vi "set stage speeds.vi"() -> ()   [LabVIEW 2012]
uses:
  GFG/GFGnumericGet.vi
  GFG/GFG library.lvlib
panel:
  in  "fast":dbl
  in  "slow":dbl
  in  "OK Button":bool
  # "Set stage speed (arbitrary units)"
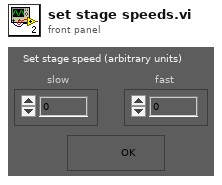
[diagram p1: front panel]
types:
  T1 = enum32{"Invalid", "Standard", "Closed", "Hidden", "Minimized", "Maximized"}
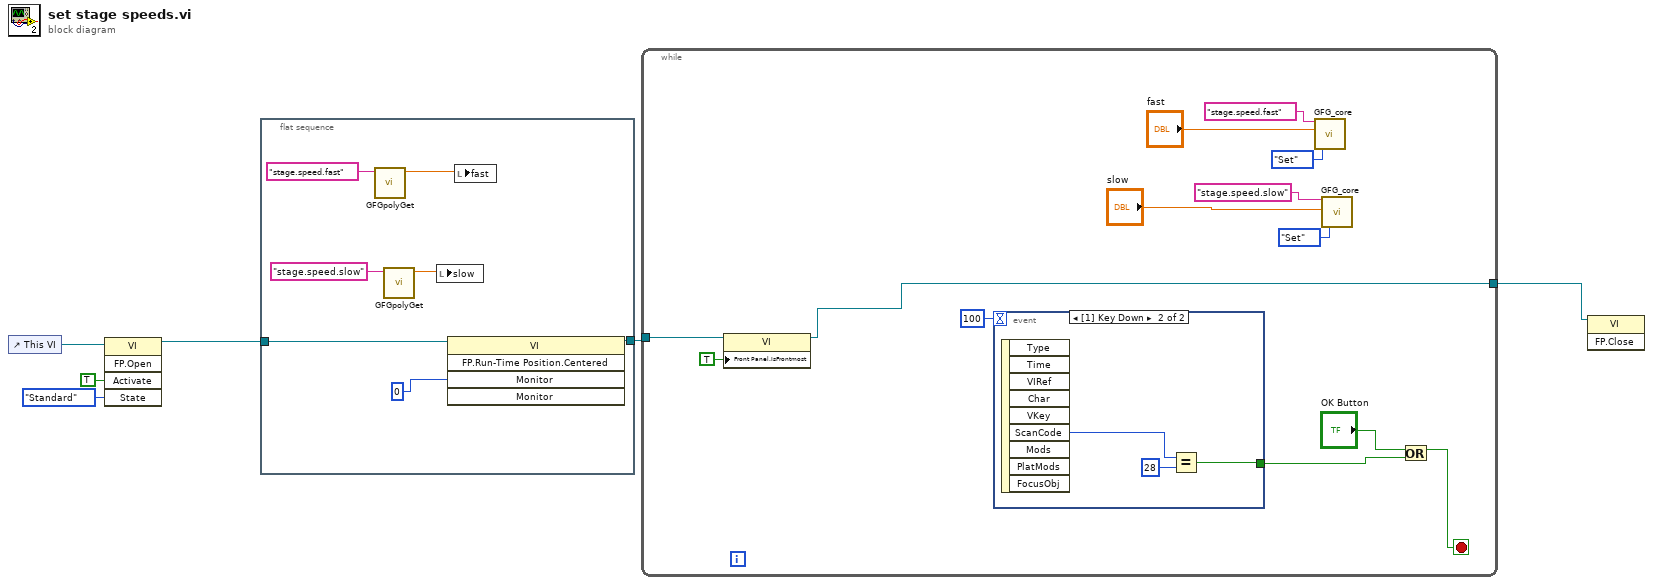
[diagram p0: block diagram]
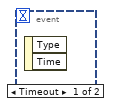
[diagram p2: hidden frame]
diagram:
  n1 = control-ref of="This VI"() -> (w4:refnum<vi>)
  n2 = invoke class="VI" method="FP.Open"(reference=w4, "Activate"=TRUE ("Activate?"), "State"=T1."Standard") -> (reference out=w1:refnum<vi>)  [unwired: 2 in, 4 out]
  n3 = flat-sequence {
    tunnel: [w12] -> w2
    tunnel: w1 -> [w11]
    frame #0 {
      n4 = call-poly "GFGpolyGet.vi"("Variable Name in"="stage.speed.fast") -> ("Numeric"=w8:dbl)  [unwired: 9 in, 1 out]
      n5 = call-poly "GFGpolyGet.vi"("Variable Name in"="stage.speed.slow") -> ("Numeric"=w7:dbl)  [unwired: 9 in, 1 out]
      n6 = local write "slow"(w7) -> ()
      n7 = invoke class="VI" method="FP.Run-Time Position.Centered"(reference=w11, "Monitor"=i16 0) -> (reference out=w12:refnum<vi>)  [unwired: 3 in, 4 out]
      n8 = local write "fast"(w8) -> ()
    }
  }
  n9 = while {
    tunnel: w2 -> [w23]
    tunnel: [w22] -> w3
    stop <- w21 stop-if-true
    n10 = property class="VI"(reference=w23, "Front Panel.IsFrontmost"=TRUE ("Front Panel Window:Is Frontmost")) -> (reference out=w22:refnum<vi>)  [unwired: 1 in, 1 out]
    n11 = event shown="[1] Key Down" {
      selector: _ -> [_ _]
      dyn-events: _ -> [_ _]
      timeout: 100 -> [_ _]
      tunnel: [_ w27] -> w20
      event Timeout {
        n12 = event-data() -> ()  [unwired: 1 in, 2 out]
      }
      event Key Down {
        n13 = event-data() -> ("ScanCode"=w29:i16)  [unwired: 1 in, 8 out]
        n14 = Equal?(x=w29, y=i16 28) -> (x = y?=w27:bool)
      }
    }
    n15 = call "GFG_core.vi"("Variable Name in"="stage.speed.fast", "Variant in"="fast", "Action"=enum16{"Init", "Set", "Get"}."Set") -> ()  [unwired: 10 in, 7 out]
    n16 = call "GFG_core.vi"("Variable Name in"="stage.speed.slow", "Variant in"="slow", "Action"=enum16{"Init", "Set", "Get"}."Set") -> ()  [unwired: 10 in, 7 out]
    n17 = Or(x="OK Button", y=w20) -> (x .or. y?=w21:bool)
  }
  n18 = invoke class="VI" method="FP.Close"(reference=w3) -> ()  [unwired: 2 in, 3 out]
